vi "RSNRPZ Set Time Slot Width.vi"(8 "error in (no error)":errorcluster, 9 "Width (1.0e-3 s)":dbl=0.001 format="%.2p", 10 "Channel (1)":i32=1, 11 "VISA session":refnum<visa-resource-name> caption="VISA resource name") -> (0 "error out":errorcluster, 3 "dup VISA session":refnum<visa-resource-name> caption="VISA resource name")   [LabVIEW 2010]
doc: "This VI sets the length of the timeslot in the Timeslot mode.\n\nNote:\n\n1) This VI is not available for NRP-Z51.\n\nRemote-control command(s):\nSENS:POW:TSL:AVG:WIDT"
uses:
  rsnrpz_32.dll
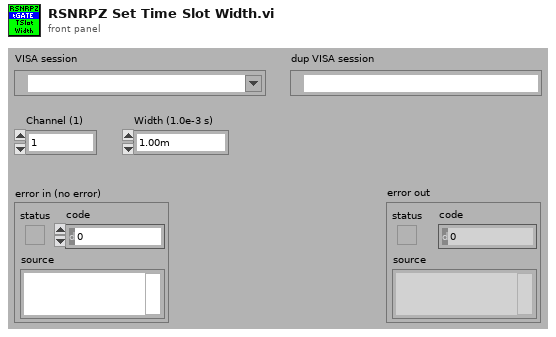
[diagram p1: front panel]
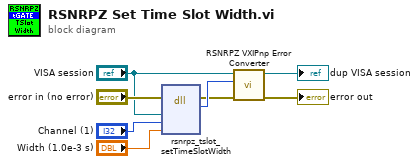
[diagram p0: block diagram]
diagram:
  n1 = dll-call lib="rsnrpz_32.dll" fn="rsnrpz_tslot_setTimeSlotWidth"(error in="error in (no error)", "VISA Session"="VISA session", "Channel"="Channel (1)", "Width"="Width (1.0e-3 s)") -> (error out=w5:errorcluster, "Status"=w8:i32)  [unwired: 5 in, 1 out]
  n2 = call <instrlib>:"RSNRPZ VXIPnp Error Converter.vi"("error in"=w5, "VXIPnp error code"=w8, "VISA session"="VISA session") -> ("error out"=→"error out":errorcluster, "dup VISA session"=→"dup VISA session":refnum<visa-resource-name>)  [unwired: 7 in]
